vi "Demo.vi"() -> ()   [LabVIEW 2016, in "XControl Custom Time Display.xctl"]
uses:
  XControl Custom Time Display.xctl
panel:
  out "XControl Custom Time Display":dbl(xcontrol)
  in  "milliseconds to wait":u32=20
  in  "Stop Button":bool
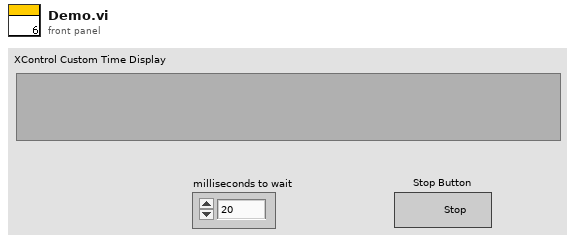
[diagram p1: front panel]
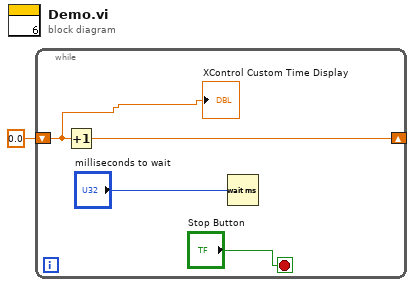
[diagram p0: block diagram]
diagram:
  n1 = while {
    shift-right: [w3] -> _
    shift-left: 0.0 -> [w2]
    stop <- "Stop Button" stop-if-true
    n2 = Increment(x=w2) -> (x+1=w3:dbl)
    n3 = Wait (ms)(milliseconds to wait="milliseconds to wait") -> ()  [unwired: 1 out]
    "XControl Custom Time Display" <- w2
  }
